vi "NavX Background Loop.vi"() -> ()   [LabVIEW 2015]
uses:
  Support/Global Objects.vi
  navX Library v2/navX Library v2.lvlib
panel:
  out "Roll":dbl
  out "Pitch":dbl
  out "Yaw":dbl
  out "heading":dbl
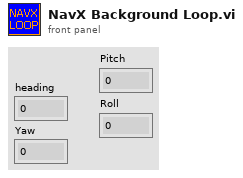
[diagram p1: front panel]
types:
  T1 = typedef "NaxX Info.ctl" = cluster{"navX Device":T2, "Current Yaw":dbl, "Active":bool, "Current Roll":dbl}
  T2 = typedef "navX Library v2.lvlib/Z900_navX_DeviceTypeDef.ctl" = cluster{"Interface":cluster{"Protocol":T3, "Update Rate (4Hz-60Hz)":u8, "navX Open TypeDef":variant}, "Notify Packet":refnum<notifier>, "Loop VI Refnum":refnum<vi>, "Ready to Close Occurrence Refnum":refnum<k4>}
  T3 = typedef "navX Library v2.lvlib/Z900_navX_ProtocolTypeDef.ctl" = enum16{"SERIAL", "I2C", "SPI"}
  T4 = cluster{"Yaw":dbl, "Roll":dbl, "Pitch":dbl, "Heading":dbl, "Fused Heading":dbl}
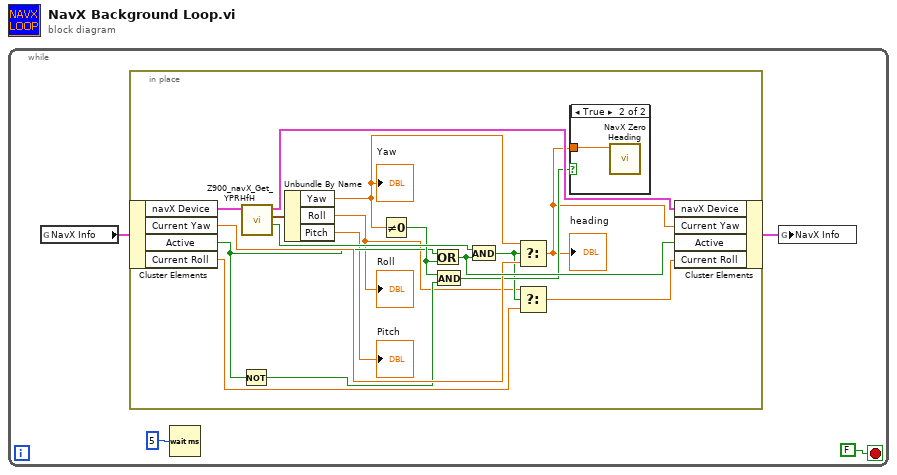
[diagram p0: block diagram]
diagram:
  n1 = while {
    stop <- FALSE stop-if-true
    n2 = global read "Global Objects.vi" "NavX Info"() -> (w4:T1)
    n3 = in-place {
      n4 = in-place-cluster #1(w4) -> ("navX Device"=w21:T2, "Current Yaw"=w16:dbl, "Active"=w13:bool, "Current Roll"=w7:dbl)
      n5 = Not(x=w13) -> (.not. x?=w14:bool)
      n6 = call "Z900_navX_Get_YPRHfH.vi"("navX Device"=w21) -> ("Connected"=w17:bool, "YRPHfH"=w19:T4, "navX Device"=w20:T2)  [unwired: 7 in, 1 out]
      n7 = Unbundle By Name(w19) -> ("Yaw"=w10:dbl, "Roll"=w6:dbl, "Pitch"=→"Pitch":dbl)
      "Yaw" <- w10
      "Roll" <- w6
      n8 = Not Equal To 0?(x=w10) -> (x != 0?=w15:bool)
      n9 = Or(x=w13, y=w15) -> (x .or. y?=w18:bool)
      n10 = And(x=w15, y=w14) -> (x .and. y?=w12:bool)
      n11 = And(x=w17, y=w18) -> (x .and. y?=w8:bool)
      n12 = Select(t=w10, s=w8, f=w16) -> (s? t:f=w11:dbl)
      "heading" <- w11
      n13 = Select(t=w6, s=w8, f=w7) -> (s? t:f=w5:dbl)
      n14 = case shown="True" w12 {
        tunnel: w11 -> [_ w22]
        frame False {
        }
        frame True {
          n15 = call "NavX Zero Heading.vi"("Default Heading"=w22) -> ()  [unwired: 10 in, 1 out]
        }
      }
      n16 = in-place-cluster #1("navX Device"=w20, "Current Yaw"=w11, "Active"=w18, "Current Roll"=w5) -> (w1:T1)
    }
    n17 = Wait (ms)(milliseconds to wait=u32 5) -> ()  [unwired: 1 out]
    n18 = global write "Global Objects.vi" "NavX Info"(w1) -> ()
  }
